vi "Set State.vi"(8 "error in (no error)":errorcluster, 10 "State":T1, 11 "Panel in":refnum<class "Panel.lvclass">) -> (0 "error out":errorcluster, 3 "Panel out":refnum<class "Panel.lvclass">)   [LabVIEW 2018, in "OOPanel.lvlib" / "Panel.lvclass"]
uses:
  Panel.lvclass
  State.ctl
  Panel.lvclass/Panel.ctl
  Panel Visibility Changed.ctl
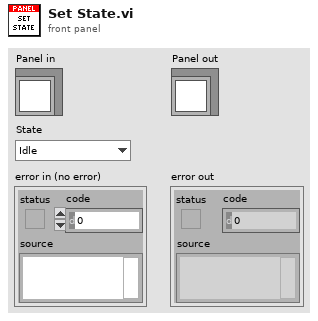
[diagram p1: front panel]
types:
  T1 = typedef "OOPanel.lvlib/Panel.lvclass/State.ctl" = enum16{"Idle", "Hidden", "Visible", "Subpanel"}
  T2 = typedef "OOPanel.lvlib/Panel.lvclass/Panel Visibility Changed.ctl" = cluster{"State":T1}
  T3 = typedef "OOPanel.lvlib/Panel.lvclass/Ref Data.ctl" = cluster{"Panel VI":refnum<vi>, "Close":bool, "Panel Events":T4, "Running":bool, "Desired Size":T5, "Subpanel":refnum<vi>, "State":T1}
  T4 = typedef "OOPanel.lvlib/Panel.lvclass/Panel Events.ctl" = cluster{"Close":refnum<user-event>, "Visibility Changed":refnum<user-event>}
  T5 = typedef "OOPanel.lvlib/Panel.lvclass/Desired Size.ctl" = cluster{"Width":i16, "Height":i16}
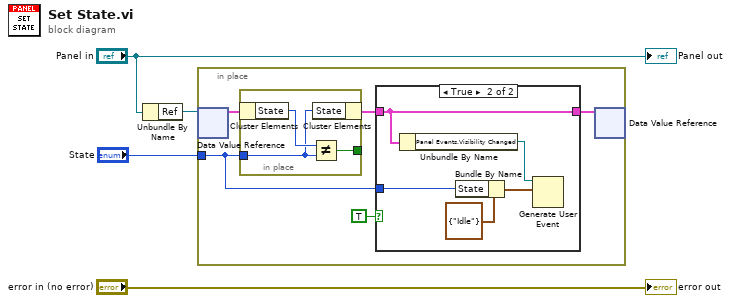
[diagram p0: block diagram]
diagram:
  n1 = Unbundle By Name("Panel in") -> ("Ref"=w3:refnum<data-value>)
  n2 = in-place {
    in-place-border: "State" -> [w7]
    n3 = in-place-dvr #1(w3) -> (w9:T3)  [unwired: 1 out]
    n4 = in-place {
      in-place-border: w7 -> [w17]
      in-place-border: [w16] -> _
      n5 = in-place-cluster #2(w9) -> ("State"=w18:T1)
      n6 = Not Equal?(x=w18, y=w17) -> (x != y?=w16:bool)
      n7 = in-place-cluster #2("State"=w17) -> (w8:T3)
    }
    n8 = case shown="True" TRUE {
      tunnel: w8 -> [w10 w11]
      tunnel: w7 -> [_ w13]
      tunnel: [w10 w11] -> w6
      frame False {
      }
      frame True {
        n9 = Unbundle By Name(w11) -> ("Panel Events.Visibility Changed"=w15:refnum<user-event>)
        n10 = Bundle By Name(cluster=T2 {"State"=enum."Idle"} ("Panel Visibility Changed"), "State"=w13) -> (w12:T2)
        n11 = Generate User Event(user event=w15, event data cluster=w12) -> ()  [unwired: 2 in, 2 out]
      }
    }
    n12 = in-place-dvr #1(w6) -> ()  [unwired: 2 out]
  }
  "error out" <- "error in (no error)"
  "Panel out" <- "Panel in"
